vi "CAN FD.vi"() -> ()   [LabVIEW 2022 SP3]
uses:
  <vilib>/xnet/xnet.llb/XNET Frame CAN.ctl
  <vilib>/xnet/xnet.llb/XNET Frame Type CAN.ctl
  <vilib>/xnet/xnet.llb/XNET Create Session (Frame Output Queued).vi
  <vilib>/xnet/xnet.llb/XNET Write (Frame CAN).vi
  <vilib>/xnet/xnet.llb/XNET Create Session (Frame Input Stream).vi
  <vilib>/xnet/xnet.llb/XNET Read (Frame CAN).vi
  <resource>/objmgr/xnet.rc
panel:
  out "Interface:CAN:I/O Mode 2":u32(ring) items=["CAN 2.0", "CAN FD", "CAN FD+BRS"]
  in  "stop 2":bool
  out "Frames":string[][](table)=[["2018/11/30 15:51:31", "00\r\n", "00000600", "CAN Remote", "No", "No"], ["2018/11/30 15:51:31", "00\t00\t00\t00\t00\t00\t00\r\n", "00000465", "CAN Remote", "No", "No"], ["2018/11/30 15:51:31", "24\t37\t5C\t0C\t72\tFA\t57\r\n", "00000159", "CAN Data", "No", "No"], ["", "", "", "", "", ""], ["", "", "", "", "", ""], ["", "", "", "", "", ""], ["", "", "", "", "", ""], ["", "", "", "", "", ""], ["", "", "", "", "", ""], ["", "", "", "", "", ""], ["", "", "", "", "", ""], ["", "", "", "", "", ""], ["", "", "", "", "", ""], ["", "", "", "", "", ""], ["", "", "", "", "", ""]]
  in  "Hex Display":bool=TRUE
  in  "Number of Frames to Display":i32=15
  in  "stop":bool
  in  "Select Interface":refnum<k21>="CAN1"
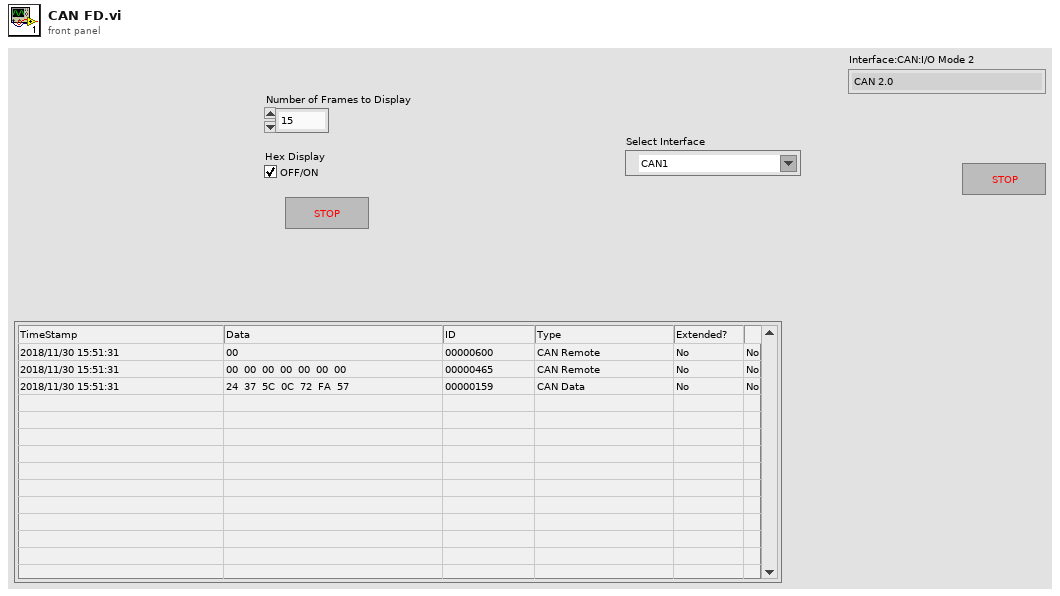
[diagram p1: front panel]
types:
  T1 = typedef "XNET Frame CAN.ctl" = cluster{"timestamp":timestamp, "payload":u8[], "identifier":u32, "type":T2, "extended?":bool, "echo?":bool}
  T2 = typedef "XNET Frame Type CAN.ctl" = u8
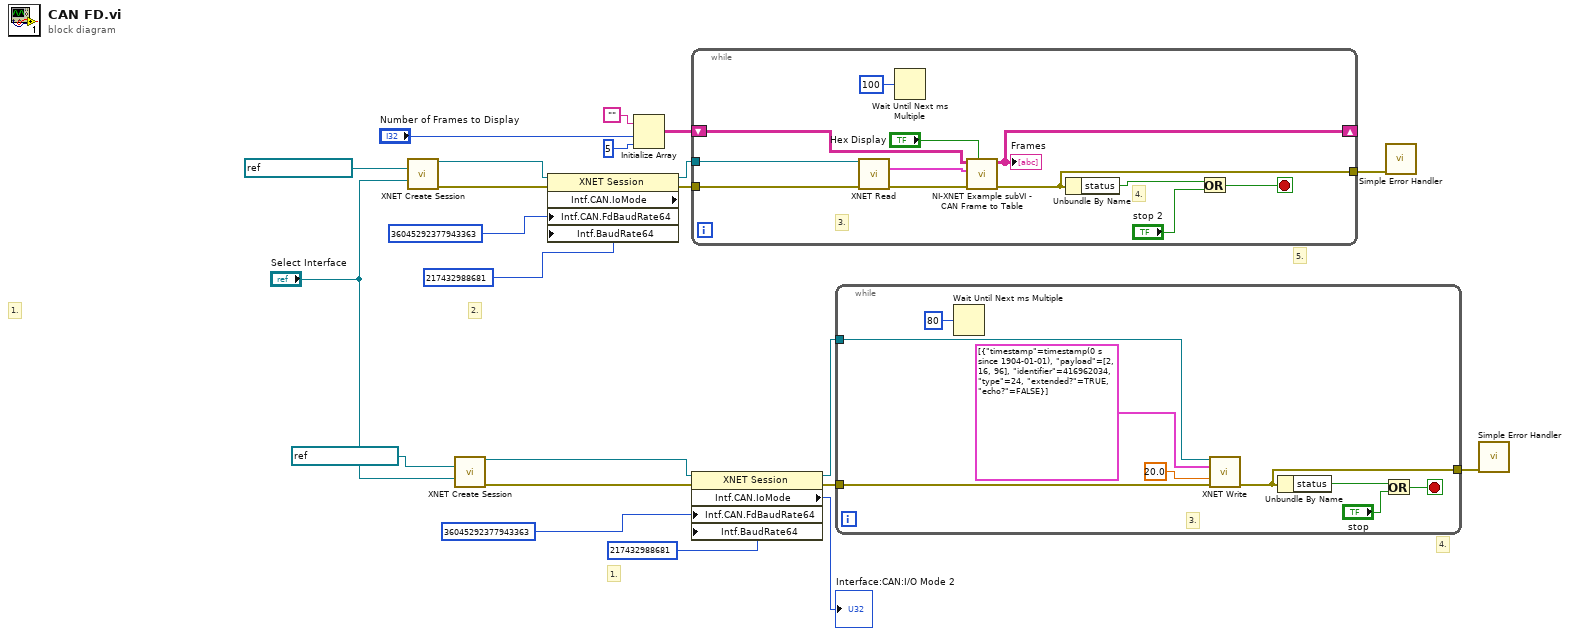
[diagram p0: block diagram]
diagram:
  # "2."
  # "5."
  # "1."
  # "4."
  # "1."
  n1 = call-poly <vilib>:"XNET Create Session.vi"("cluster (:memory:)"=refnum<k21> "Elatch_Labview", "interface"="Select Interface") -> ("session out"=w8:refnum<k21>, "error out"=w6:errorcluster)  [unwired: 1 in, 11 out]
  n2 = call-poly <vilib>:"XNET Create Session.vi"("frame"=refnum<k21> "Escritura\nElatch_Labview", "interface"="Select Interface") -> ("session out"=w10:refnum<k21>, "error out"=w15:errorcluster)  [unwired: 1 in, 11 out]
  n3 = property class="XNET Session" props=["Intf.CAN.IoMode", "Intf.CAN.FdBaudRate64", "Intf.BaudRate64"](reference=w8, error in=w6, "Intf.CAN.FdBaudRate64"=u64 36045292377943363 ("Interface:CAN:64bit FD Baud Rate"), "Intf.BaudRate64"=u64 217432988681 ("Interface:64bit Baud Rate")) -> (reference out=w7:refnum<k21>, error out=w5:errorcluster)  [unwired: 1 out]
  n4 = Initialize Array("", "Number of Frames to Display", 5 ("Dimension Size")) -> (w17:string[][])
  n5 = while {
    tunnel: w7 -> [w34]
    tunnel: w5 -> [w33]
    tunnel: [w25] -> w21
    shift-right: [w27] -> _
    shift-left: w17 -> [w29]
    stop <- w30 stop-if-true
    # "4."
    # "3."
    n6 = call-poly <vilib>:"XNET Read.vi"("session in"=w34, "error in (no error)"=w33) -> ("data"=w28:T1[], "error out"=w26:errorcluster)  [unwired: 12 out]
    n7 = Wait Until Next ms Multiple(millisecond multiple=u32 100 ("milliseconds to wait")) -> ()  [unwired: 1 out]
    n8 = call "NI-XNET Example subVI - CAN Frame to Table.vi"("Hexadecimal?"="Hex Display", "error in (no error)"=w26, "CAN Frames (from XNET Read)"=w28, "Input Array"=w29) -> ("error out"=w25:errorcluster, "Output Array"=w27:string[][])  [unwired: 1 in, 5 out]
    "Frames" <- w27
    n9 = Unbundle By Name(w25) -> ("status"=w32:bool)
    n10 = Or(x=w32, y="stop 2") -> (x .or. y?=w30:bool)
  }
  n11 = property class="XNET Session"(reference=w10, error in=w15, "Intf.CAN.FdBaudRate64"=u64 36045292377943363 ("Interface:CAN:64bit FD Baud Rate"), "Intf.BaudRate64"=u64 217432988681 ("Interface:64bit Baud Rate")) -> (reference out=w12:refnum<k21>, error out=w11:errorcluster, "Intf.CAN.IoMode"=→"Interface:CAN:I/O Mode 2":u32)
  n12 = while {
    tunnel: [w40] -> w22
    tunnel: w12 -> [w37]
    tunnel: w11 -> [w36]
    stop <- w42 stop-if-true
    # "3."
    n13 = Wait Until Next ms Multiple(millisecond multiple=u32 80 ("milliseconds to wait")) -> ()  [unwired: 1 out]
    n14 = call-poly <vilib>:"XNET Write.vi"("session in"=w37, "data"=T1[] [{"timestamp"=timestamp(0 s since 1904-01-01), "payload"=[2, 16, 96], "identifier"=416962034, "type"=24, "extended?"=TRUE, "echo?"=FALSE}], "timeout (10)"=20.0, "error in (no error)"=w36) -> ("error out"=w40:errorcluster)  [unwired: 11 out]
    n15 = Unbundle By Name(w40) -> ("status"=w41:bool)
    n16 = Or(x=w41, y="stop") -> (x .or. y?=w42:bool)
  }
  n17 = call <vilib>:"Simple Error Handler.vi"("error in (no error)"=w21) -> ()  [unwired: 1 in, 8 out]
  n18 = call <vilib>:"Simple Error Handler.vi"("error in (no error)"=w22) -> ()  [unwired: 1 in, 8 out]
